vi "test_pubsub.vi"() -> ()   [LabVIEW 2010]
panel:
  out "equal send":bool
  out "equal receive":bool
  in  "npub":i32=3
  in  "nsub":i32=2
  out "success?":bool
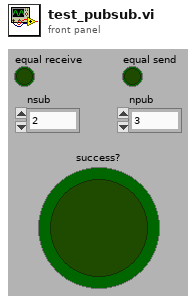
[diagram p1: front panel]
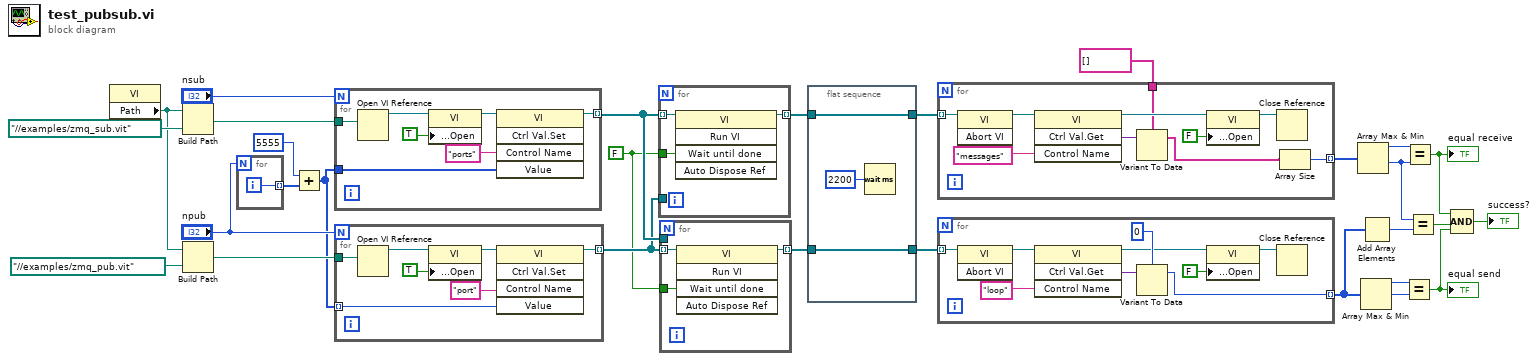
[diagram p0: block diagram]
diagram:
  w12 = FALSE
  n1 = property class="VI"() -> ("Path"=w27:path)  [unwired: 2 in, 2 out]
  n2 = Build Path(base path=w27, name or relative path=path "../../examples/zmq_sub.vit" ("VI Path")) -> (appended path=w26:path)
  n3 = Build Path(base path=w27, name or relative path=path "../../examples/zmq_pub.vit" ("VI Path")) -> (appended path=w24:path)
  n4 = for {
    N: "npub" -> [_]
    tunnel: [w30] -> w19 mode=indexing
    i -> [w30]
  }
  n5 = Add(x=5555, y=w19) -> (x+y=w17:i32[])
  n6 = for {
    N: "nsub" -> [_]
    tunnel: [w31] -> w14 mode=indexing
    tunnel: w26 -> [w35]
    tunnel: w17 -> [w33]
    n7 = Open VI Reference(vi path=w35) -> (vi reference=w37:refnum<vi>)  [unwired: 5 in, 1 out]
    n8 = property class="VI"(reference=w37, "Front Panel.Open"=TRUE ("Front Panel Window:Open")) -> (reference out=w34:refnum<vi>)  [unwired: 1 in, 1 out]
    n9 = invoke class="VI" method="Ctrl Val.Set"(reference=w34, "Control Name"="ports", "Value"=w33) -> (reference out=w31:refnum<vi>)  [unwired: 2 in, 4 out]
  }
  n10 = for {
    N: "npub" -> [_]
    tunnel: [w38] -> w13 mode=indexing
    tunnel: w24 -> [w40]
    tunnel: w17 -> [w39] mode=indexing
    n11 = Open VI Reference(vi path=w40) -> (vi reference=w42:refnum<vi>)  [unwired: 5 in, 1 out]
    n12 = property class="VI"(reference=w42, "Front Panel.Open"=TRUE ("Front Panel Window:Open")) -> (reference out=w43:refnum<vi>)  [unwired: 1 in, 1 out]
    n13 = invoke class="VI" method="Ctrl Val.Set"(reference=w43, "Control Name"="port", "Value"=w39) -> (reference out=w38:refnum<vi>)  [unwired: 2 in, 4 out]
  }
  n14 = for {
    tunnel: [w47] -> w16 mode=indexing
    tunnel: w14 -> [w46] mode=indexing
    tunnel: w13 -> [_]
    tunnel: w12 -> [w45]
    n15 = invoke class="VI" method="Run VI"(reference=w46, "Wait until done"=w45) -> (reference out=w47:refnum<vi>)  [unwired: 3 in, 4 out]
  }
  n16 = for {
    tunnel: [w50] -> w15 mode=indexing
    tunnel: w13 -> [w49] mode=indexing
    tunnel: w14 -> [_]
    tunnel: w12 -> [w48]
    n17 = invoke class="VI" method="Run VI"(reference=w49, "Wait until done"=w48) -> (reference out=w50:refnum<vi>)  [unwired: 3 in, 4 out]
  }
  n18 = flat-sequence {
    tunnel: w15 -> [w52]
    tunnel: w16 -> [w51]
    tunnel: [w52] -> w25
    tunnel: [w51] -> w23
    frame #0 {
      n19 = Wait (ms)(milliseconds to wait=u32 2200) -> ()  [unwired: 1 out]
    }
  }
  n20 = for {
    tunnel: w23 -> [w63] mode=indexing
    tunnel: string[] [] -> [w56]
    tunnel: [w54] -> w11 mode=indexing
    n21 = invoke class="VI" method="Abort VI"(reference=w63) -> (reference out=w62:refnum<vi>)  [unwired: 2 in, 2 out]
    n22 = invoke class="VI" method="Ctrl Val.Get"(reference=w62, "Control Name"="messages") -> (reference out=w58:refnum<vi>, "Get Control Value Variant"=w60:variant)  [unwired: 2 in, 2 out]
    n23 = Variant To Data(Variant=w60, type=w56) -> (data=w55:string[])  [unwired: 1 in, 1 out]
    n24 = property class="VI"(reference=w58, "Front Panel.Open"=FALSE ("Front Panel Window:Open")) -> (reference out=w59:refnum<vi>)  [unwired: 1 in, 1 out]
    n25 = Close Reference(reference=w59) -> ()  [unwired: 1 in, 1 out]
    n26 = Array Size(array=w55) -> (size(s)=w54:i32)
  }
  n27 = for {
    tunnel: w25 -> [w72] mode=indexing
    tunnel: [w64] -> w2 mode=indexing
    n28 = invoke class="VI" method="Abort VI"(reference=w72) -> (reference out=w71:refnum<vi>)  [unwired: 2 in, 2 out]
    n29 = invoke class="VI" method="Ctrl Val.Get"(reference=w71, "Control Name"="loop") -> (reference out=w66:refnum<vi>, "Get Control Value Variant"=w69:variant)  [unwired: 2 in, 2 out]
    n30 = Variant To Data(Variant=w69, type=0) -> (data=w64:i32)  [unwired: 1 in, 1 out]
    n31 = property class="VI"(reference=w66, "Front Panel.Open"=FALSE ("Front Panel Window:Open")) -> (reference out=w67:refnum<vi>)  [unwired: 1 in, 1 out]
    n32 = Close Reference(reference=w67) -> ()  [unwired: 1 in, 1 out]
  }
  n33 = Array Max & Min(array=w11) -> (max value=w10:i32, min value=w8:i32)  [unwired: 2 out]
  n34 = Array Max & Min(array=w2) -> (max value=w7:i32, min value=w9:i32)  [unwired: 2 out]
  n35 = Add Array Elements(numeric array=w2) -> (sum=w1:i32)
  n36 = Equal?(x=w7, y=w9) -> (x = y?=w6:bool)
  "equal send" <- w6
  n37 = Equal?(x=w10, y=w8) -> (x = y?=w4:bool)
  "equal receive" <- w4
  n38 = Equal?(x=w8, y=w1) -> (x = y?=w5:bool)
  n39 = Compound Arithmetic op=AND(w4, w5, w6) -> (→"success?":bool)
